vi "Agilent VNA Read Number of Available Traces.vi"(7 "Agilent VNA":T1, 8 "error in (no error)":errorcluster, 11 "VISA Resource Name":refnum<visa-resource-name>) -> (0 "error out":errorcluster, 2 "Number of Traces":i8, 3 "dup VISA Resource Name":refnum<visa-resource-name>)   [LabVIEW 2011]
doc: "This VI for the HP 8753 is used to read the sweep type.\n\n0 LINEAR FREQ\n1 LOG FREQ\n2 LIST FREQ\n3 CW TIME\n4 POWER SWEEP"
uses:
  TypeDefs/Agilent VNA Instrument Info.ctl
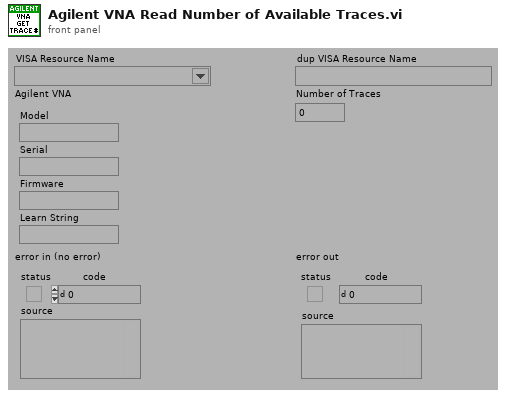
[diagram p1: front panel]
types:
  T1 = typedef "Agilent VNA Instrument Info.ctl" = cluster{"Model":string, "Serial":string, "Firmware":string, "Learn String":string}
  T2 = typedef "Agilent VNA Model.ctl" = enum16{"Not Supported", "8510X", "8719X", "8720X", "8722X", "8753X", "ENA", "PNA", "Field Fox"}
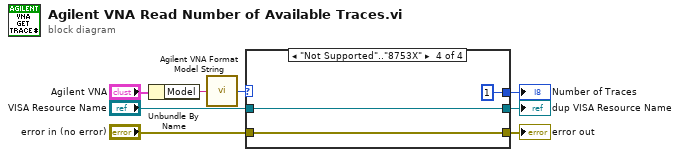
[diagram p0: block diagram]
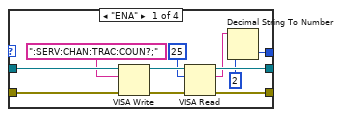
[diagram p2: hidden frame]
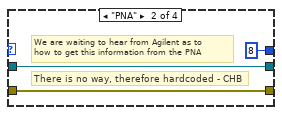
[diagram p3: hidden frame]
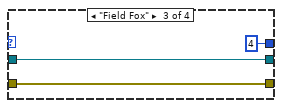
[diagram p4: hidden frame]
diagram:
  n1 = Unbundle By Name("Agilent VNA") -> ("Model"=w1:string)
  n2 = call "Agilent VNA Format Model String.vi"("Model"=w1) -> ("Model"=w3:T2)
  n3 = case shown="\"Not Supported\"..\"8753X\"" w3 {
    tunnel: "VISA Resource Name" -> [w15 w22 w25 w27]
    tunnel: "error in (no error)" -> [w19 w21 w24 w28]
    tunnel: [w18 w21 w24 w28] -> w7
    tunnel: [w10 i8 8 ("Number of Channels") i8 4 ("Number of Channels") i8 1] -> w6
    tunnel: [w13 w22 w25 w27] -> w4
    frame "ENA" {
      n4 = VISA Write(VISA resource name=w15, write buffer=":SERV:CHAN:TRAC:COUN?;", error in (no error)=w19) -> (VISA resource name out=w16:refnum<visa-resource-name>, error out=w17:errorcluster)  [unwired: 1 out]
      n5 = VISA Read(VISA resource name=w16, byte count=u32 25, error in (no error)=w17) -> (VISA resource name out=w13:refnum<visa-resource-name>, read buffer=w12:string, error out=w18:errorcluster)  [unwired: 1 out]
      n6 = Decimal String To Number(string=w12, default (0L)=i8 2 ("Number of Channels")) -> (number=w10:i8)  [unwired: 2 out]
    }
    frame "PNA" {
      # "There is no way, therefore hardcoded - CHB"
      # "We are waiting to hear from Agilent as to\nhow to get this information from the PNA"
    }
    frame "Field Fox" {
    }
    frame "Not Supported".."8753X" {
    }
  }
  "Number of Traces" <- w6
  "dup VISA Resource Name" <- w4
  "error out" <- w7
